vi "PLC SImulation.vi"() -> ()   [LabVIEW 2017]
panel:
  in  "stop":bool
  # "PLC Simulation"
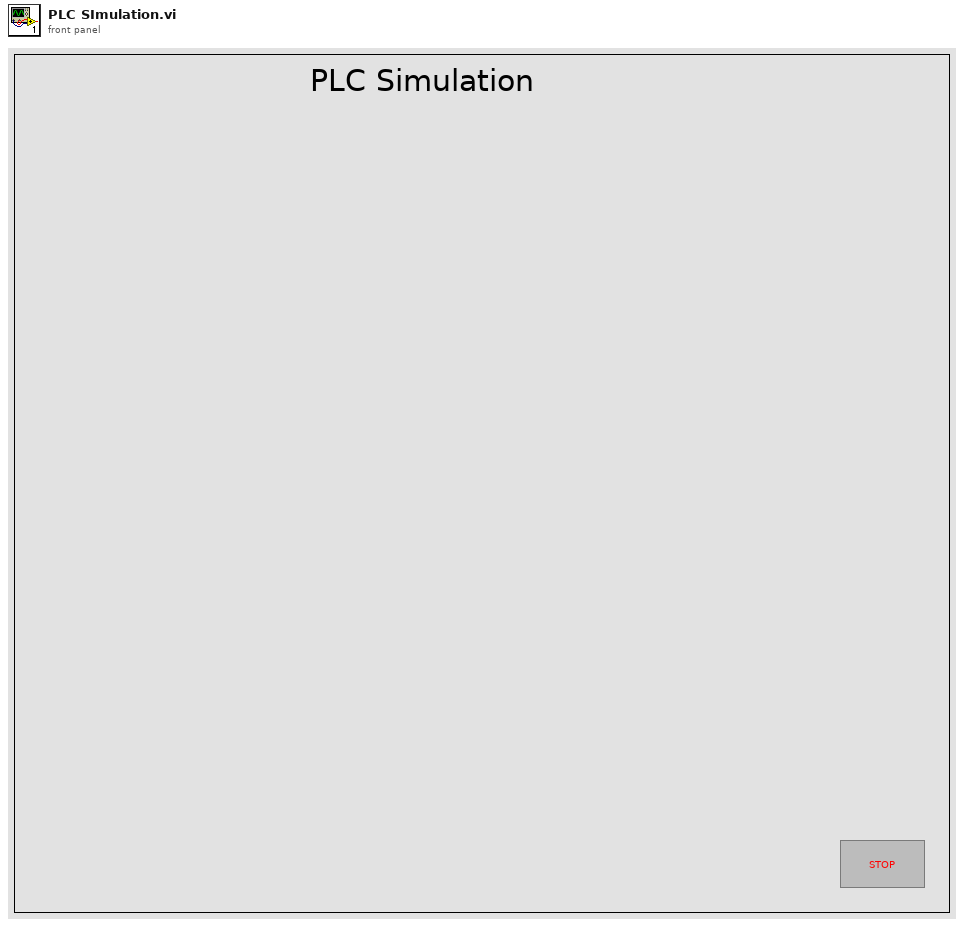
[diagram p1: front panel]
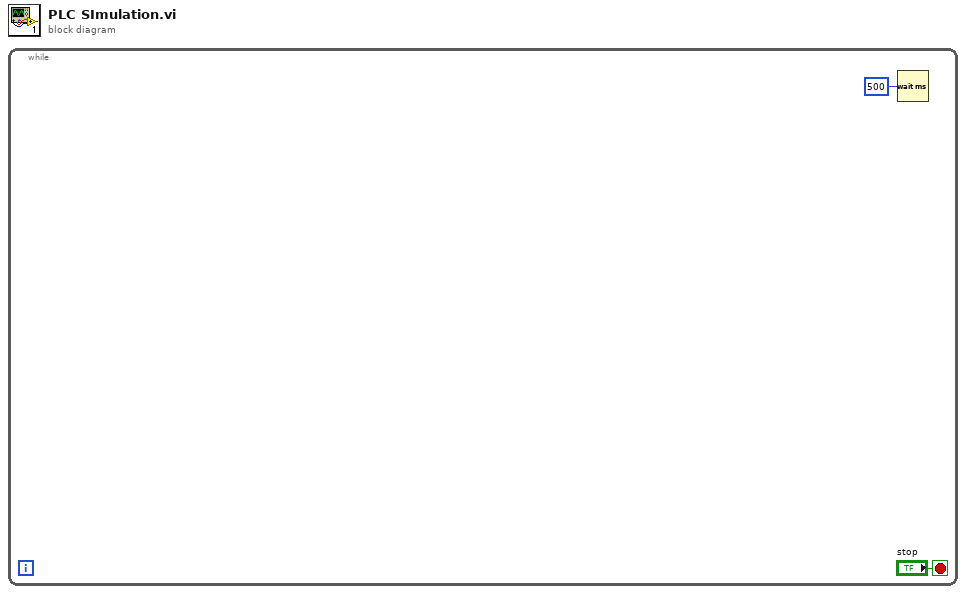
[diagram p0: block diagram]
diagram:
  n1 = while {
    stop <- "stop" stop-if-true
    n2 = Wait (ms)(milliseconds to wait=u32 500) -> ()  [unwired: 1 out]
  }
